vi "queues3.vi"() -> ()   [LabVIEW 2019]
doc: "This is the first of two demos using Queues. In this demo, one While loop takes the same role as the first loop in the Notifier example, whilst the second While loop plots data. Here, however, the Wait period in the second (consumer) loop is longer than the producer, and so data builds up over time. Because these are using a Queue, the data is not lost - it merely becomes backlogged."
panel:
  out "Sum":i32
  out "Consumer 2":i32
  out "Waveform Chart 2":dbl(graph)
  out "Consumer1":i32
  out "Producer":i32
  in  "stop":bool
  out "Waveform Chart":dbl(graph)
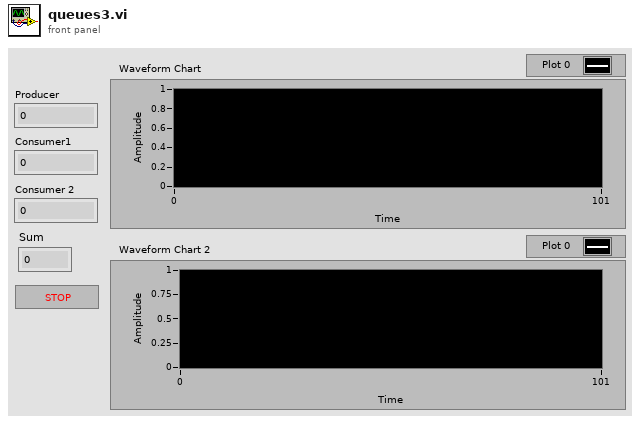
[diagram p1: front panel]
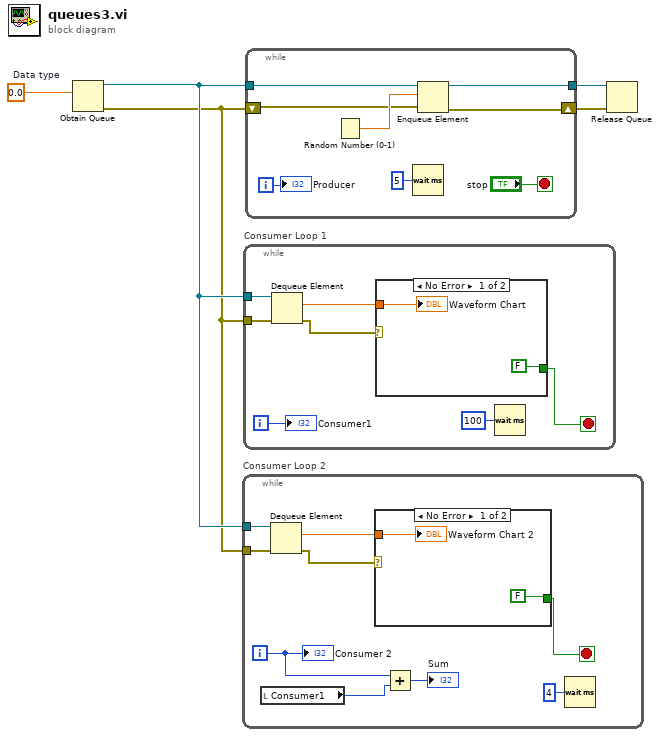
[diagram p0: block diagram]
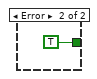
[diagram p2: hidden frame]
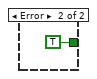
[diagram p3: hidden frame]
diagram:
  w5 = 0.0  # Data type
  n1 = Obtain Queue(element data type=w5) -> (queue out=w2:refnum<queue>, error out=w1:errorcluster)  [unwired: 4 in, 1 out]
  n2 = while "Consumer Loop 2" {
    tunnel: w2 -> [w14]
    tunnel: w1 -> [w10]
    i -> [w8]
    stop <- w11 stop-if-true
    n3 = local read "Consumer1"() -> (w9:i32)
    n4 = Dequeue Element(queue=w14, error in (no error)=w10) -> (element=w12:dbl, error out=w13:errorcluster)  [unwired: 1 in, 2 out]
    n5 = case shown="No Error" w13 {
      tunnel: w12 -> [w16 _]
      tunnel: [FALSE TRUE] -> w11
      frame No Error {
        "Waveform Chart 2" <- w16
      }
      frame Error {
      }
    }
    n6 = Add(x=w8, y=w9) -> (x+y=→"Sum":i32)
    n7 = Wait (ms)(milliseconds to wait=u32 4) -> ()  [unwired: 1 out]
    "Consumer 2" <- w8
  }
  n8 = while "Consumer Loop 1" {
    tunnel: w2 -> [w24]
    tunnel: w1 -> [w19]
    i -> [w23]
    stop <- w20 stop-if-true
    n9 = Dequeue Element(queue=w24, error in (no error)=w19) -> (element=w21:dbl, error out=w22:errorcluster)  [unwired: 1 in, 2 out]
    n10 = case shown="No Error" w22 {
      tunnel: w21 -> [w26 _]
      tunnel: [FALSE TRUE] -> w20
      frame No Error {
        "Waveform Chart" <- w26
      }
      frame Error {
      }
    }
    n11 = Wait (ms)(milliseconds to wait=u32 100) -> ()  [unwired: 1 out]
    "Consumer1" <- w23
  }
  n12 = while {
    tunnel: w2 -> [w35]
    shift-right: [w29] -> w3
    shift-left: w1 -> [w30]
    tunnel: [w28] -> w4
    i -> [w33]
    stop <- "stop" stop-if-true
    n13 = Random Number (0-1)() -> (number: 0 to 1=w31:dbl)
    n14 = Wait (ms)(milliseconds to wait=u32 5) -> ()  [unwired: 1 out]
    n15 = Enqueue Element(queue=w35, element=w31, error in (no error)=w30) -> (queue out=w28:refnum<queue>, error out=w29:errorcluster)  [unwired: 1 in, 1 out]
    "Producer" <- w33
  }
  n16 = Release Queue(queue=w4, error in (no error)=w3) -> ()  [unwired: 1 in, 3 out]
